vi "sava-4.vi"(7 "datafile":path[](array[path]), 10 "1D array":i16[](array[numeric]) caption="一维数组-2") -> ()   [LabVIEW 2012]
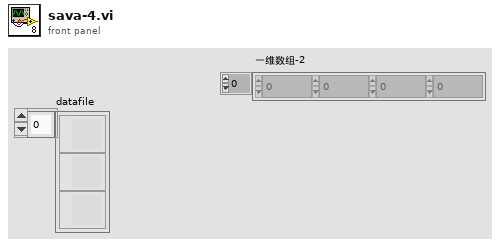
[diagram p1: front panel]
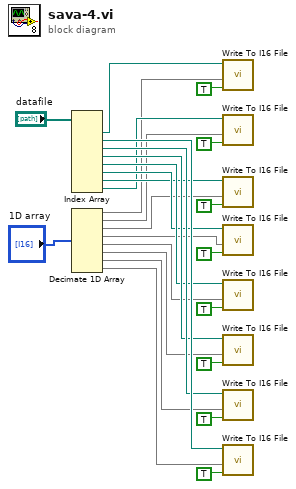
[diagram p0: block diagram]
diagram:
  n1 = Index Array(array="datafile") -> (element #1=w21:path, element #2=w20:path, element #3=w19:path, element #4=w18:path, element #5=w13:path, element #6=w12:path, element #7=w11:path, element #8=w10:path)  [unwired: 8 in]
  n2 = Decimate 1D Array("1D array") -> (w8:i16[], w7:i16[], w6:i16[], w5:i16[], w4:i16[], w3:i16[], w2:i16[], w1:i16[])
  n3 = call <vilib>:"Write To I16 File.vi"("append to file? (new file:F)"=TRUE, "1D array"=w8, "file path (dialog if empty)"=w21) -> ()  [unwired: 4 in, 1 out]
  n4 = call <vilib>:"Write To I16 File.vi"("append to file? (new file:F)"=TRUE, "1D array"=w7, "file path (dialog if empty)"=w10) -> ()  [unwired: 4 in, 1 out]
  n5 = call <vilib>:"Write To I16 File.vi"("append to file? (new file:F)"=TRUE, "1D array"=w6, "file path (dialog if empty)"=w11) -> ()  [unwired: 4 in, 1 out]
  n6 = call <vilib>:"Write To I16 File.vi"("append to file? (new file:F)"=TRUE, "1D array"=w5, "file path (dialog if empty)"=w12) -> ()  [unwired: 4 in, 1 out]
  n7 = call <vilib>:"Write To I16 File.vi"("append to file? (new file:F)"=TRUE, "1D array"=w4, "file path (dialog if empty)"=w13) -> ()  [unwired: 4 in, 1 out]
  n8 = call <vilib>:"Write To I16 File.vi"("append to file? (new file:F)"=TRUE, "1D array"=w3, "file path (dialog if empty)"=w18) -> ()  [unwired: 4 in, 1 out]
  n9 = call <vilib>:"Write To I16 File.vi"("append to file? (new file:F)"=TRUE, "1D array"=w2, "file path (dialog if empty)"=w19) -> ()  [unwired: 4 in, 1 out]
  n10 = call <vilib>:"Write To I16 File.vi"("append to file? (new file:F)"=TRUE, "1D array"=w1, "file path (dialog if empty)"=w20) -> ()  [unwired: 4 in, 1 out]
